vi "task1.vi"() -> ()   [LabVIEW 2021]
uses:
  <vilib>/Utility/file.llb/Write Delimited Spreadsheet (string).vi
  <vilib>/measure/mascope.llb/Pulse Measurements 1 chan.vi
  <vilib>/Utility/file.llb/Write Delimited Spreadsheet (DBL).vi
  <vilib>/measure/NI_MAPro.lvlib
panel:
  out "error out":errorcluster
  out "duty cycle":dbl format="%.2g"
  out "pulse duration":dbl format="%.2g"
  out "period":dbl format="%.4e"
  in  "number of samples":i32=100
  out "Waveform Graph":waveform(dbl)(graph)
  in  "distance (cm)":dbl
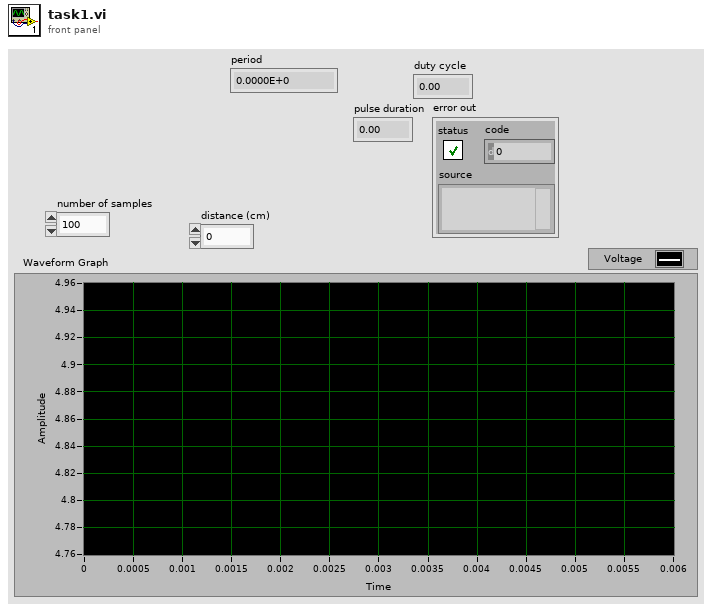
[diagram p1: front panel]
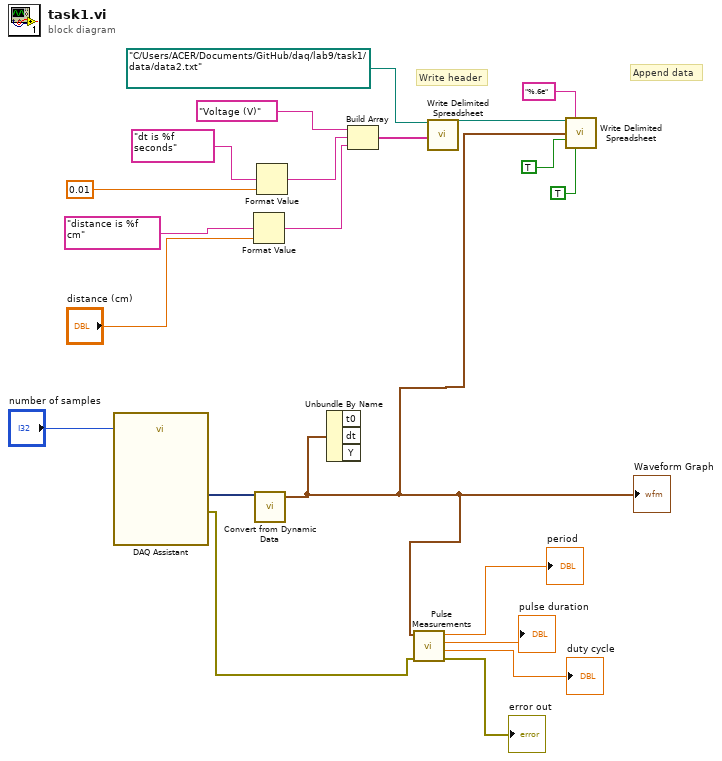
[diagram p0: block diagram]
diagram:
  # "Write header"
  # "Append data"
  n1 = call "DAQ Assistant"("number of samples"="number of samples") -> ("data"=w8:dynamicdata, "error out"=w2:errorcluster)  [unwired: 16 in, 1 out]
  n2 = Format Value(format string="distance is %f cm", value (0)="distance (cm)") -> (output string=w13:string)  [unwired: 1 in]
  n3 = call "Convert from Dynamic Data"("Dynamic Data Type"=w8) -> ("Waveform"=w1:waveform(dbl))  [unwired: 3 in]
  "Waveform Graph" <- w1
  n4 = Format Value(format string="dt is %f seconds", value (0)=0.01) -> (output string=w16:string)  [unwired: 1 in]
  n5 = Unbundle By Name(w1) -> ()  [unwired: 3 out]
  n6 = Build Array("Voltage (V)" ("element"), w16, w13) -> (w14:string[])
  n7 = call-poly <vilib>:"Pulse Measurements.vi"("error in (no error)"=w2, "signal in"=w1) -> ("error out"=→"error out":errorcluster, "duty cycle"=→"duty cycle":dbl, "pulse duration"=→"pulse duration":dbl, "period"=→"period":dbl)  [unwired: 5 in, 1 out]
  n8 = call-poly <vilib>:"Write Delimited Spreadsheet.vi"("file path (dialog if empty)"=path "C:/Users/ACER/Documents/GitHub/daq/lab9/task1/data/data2.txt", "1D data"=w14) -> ("new file path (Not A Path if cancelled)"=w20:path)  [unwired: 12 in, 1 out]
  n9 = call-poly <vilib>:"Write Delimited Spreadsheet.vi"("file path (dialog if empty)"=w20, "format (%.3f)"="%.6e", "1D data"=w1, "append to file? (new file:F)"=TRUE, "transpose? (no:F)"=TRUE) -> ()  [unwired: 9 in, 2 out]
